vi "user32_GetCapture.vi"(11 "错误输入（无错误）":errorcluster) -> (4 "hWnd":u32, 6 "success?":bool, 15 "错误输出":errorcluster)   [LabVIEW 2011]
doc: "该函数取得捕获了鼠标的窗口（如果存在）的句柄。在同一时刻，只有一个窗口能捕获鼠标；此时，该窗口接收鼠标的输入，无论光标是否在其范围内。"
uses:
  user32.dll
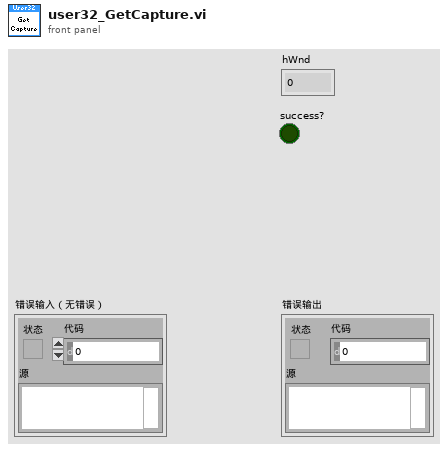
[diagram p1: front panel]
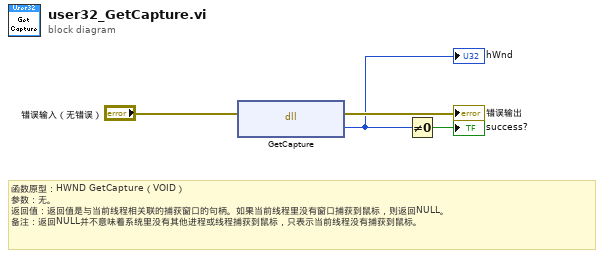
[diagram p0: block diagram]
diagram:
  # "函数原型：HWND GetCapture（VOID）\n参数：无。\n返回值：返回值是与当前线程相关联的捕获窗口的句柄。如果当前线程里没有窗口捕获到鼠标，则返回NULL。\n备注：返回NULL并不意味着系统里没有其他进程或线程捕获到鼠标，只表示当前线程没有捕获到鼠标。"
  n1 = dll-call lib="user32.dll" fn="GetCapture"(error in="错误输入（无错误）") -> (error out=→"错误输出":errorcluster, "hWnd"=w1:u32)  [unwired: 2 in, 1 out]
  "hWnd" <- w1
  n2 = Not Equal To 0?(x=w1) -> (x != 0?=→"success?":bool)
